vi "Register Test.vi"() -> (0 "error out":errorcluster, 3 "Result":bool=TRUE)   [LabVIEW 2011]
doc: "Verifies that the Registers properly store data on the CPU."
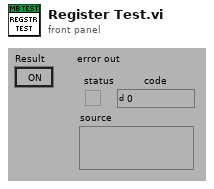
[diagram p1: front panel]
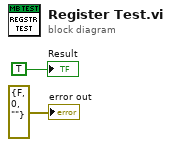
[diagram p0: block diagram]
diagram:
  "error out" <- errorcluster {"status"=FALSE, "code"=0, "source"=""} ("error out")
  "Result" <- TRUE ("PASS/FAIL Flag")
